vi "Laser Data GV.vi"() -> ()   [LabVIEW 2013]
panel:
  in  "Laser Data":i16[][][](array[numeric])
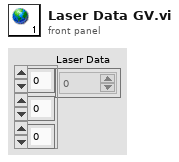
[diagram p1: front panel]
diagram:
